vi "Connect.vi"(7 "AMS":T3, 8 "Error In":errorcluster, 10 "Timeout":i32=5000, 11 "Router":string="127.0.0.1") -> (0 "Error Out":errorcluster, 1 "Device Name":string, 2 "ADS Error":T1 items=["NoError"=0, "InternalError"=1, "NoRTime"=2, "LockedMemoryError"=3, "MailBoxError"=4, "WrongHMsg"=5, "TargetPortNotFound"=6, "TargetMachineNotFound"=7, "UnknownCommandID"=8, "BadTaskID"=9, "NoIO"=10, "UnknownAmsCommand"=11, "Win32Error"=12, "PortNotConnected"=13, "InvalidAmsLength"=14, "InvalidAmsNetID"=15, "AmsSyncAmsError"=22, "AmsSyncNoIndexMap"=23, "InvalidAmsPort"=24, "NoMemory"=25, "TCPSendError"=26, "HostUnreachable"=27, "NoLockedMemory"=1280, "MailboxFull"=1282, "DeviceError"=1792, "DeviceServiceNotSupported"=1793, "DeviceInvalidGroup"=1794, "DeviceInvalidOffset"=1795, "DeviceInvalidAccess"=1796, "DeviceInvalidSize"=1797, "DeviceInvalidData"=1798, "DeviceNotReady"=1799, "DeviceBusy"=1800, "DeviceInvalidContext"=1801, "DeviceNoMemory"=1802, "DeviceInvalidParam"=1803, "DeviceNotFound"=1804, "DeviceSyntaxError"=1805, "DeviceIncompatible"=1806, "DeviceExists"=1807, "DeviceSymbolNotFound"=1808, "DeviceSymbolVersionInvalid"=1809, "DeviceInvalidState"=1810, "DeviceTransModeNotSupported"=1811, "DeviceNotifyHandleInvalid"=1812, "DeviceClientUnknown"=1813, "DeviceNoMoreHandles"=1814, "DeviceInvalidWatchsize"=1815, "DeviceNotInitialized"=1816, "DeviceTimeOut"=1817, "DeviceNoInterface"=1818, "DeviceInvalidInterface"=1819, "DeviceInvalidCLSID"=1820, "DeviceInvalidObjectID"=1821, "ClientError"=1856, "ClientInvalidParameter"=1857, "ClientListEmpty"=1858, "ClientVariableInUse"=1859, "ClientDuplicateInvokeID"=1860, "ClientSyncTimeOut"=1861, "ClientW32OR"=1862, "ClientTimeoutInvalid"=1863, "ClientPortNotOpen"=1864, "ClientNoAmsAddr"=1865, "ClientSyncInternal"=1872, "ClientAddHash"=1873, "ClientRemoveHash"=1874, "ClientNoMoreSymbols"=1875, "ClientSyncResInvalid"=1876, "ClientSyncPortLocked"=1877, "ClientQueueFull"=1878], 3 "AMS Connection":T2)   [LabVIEW 2020, in "TwinCAT ADS.lvlib"]
doc: "This connects to the <b>Router</b> (meaning any ADS server, defaults to localhost) via TCP and returns the Device Name for the <b>Target Net ID</b> and <b>Target Port</b> as well as any returned <b>ADS Error</b>. The connection may be established beside of an ADS Error."
uses:
  <userlib>/PMA/TwinCAT ADS.lvlib
  <userlib>/PMA/Low Level/TypeDefs/AMS.ctl
  <userlib>/PMA/Low Level/TypeDefs/AMS Connection.ctl
  <userlib>/PMA/Low Level/TypeDefs/ADS Error.ctl
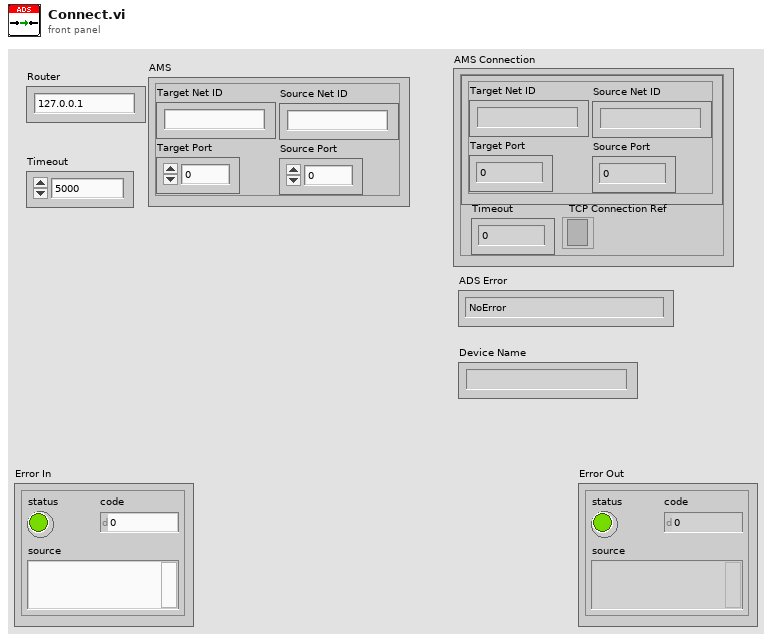
[diagram p1: front panel]
types:
  T1 = typedef "TwinCAT ADS.lvlib/ADS Error.ctl" = i32
  T2 = typedef "TwinCAT ADS.lvlib/AMS Connection.ctl" = cluster{"AMS":T3, "Timeout":i32, "TCP Connection Ref":refnum<k5>}
  T3 = typedef "TwinCAT ADS.lvlib/AMS.ctl" = cluster{"Target Net ID":string, "Target Port":u16, "Source Net ID":string, "Source Port":u16}
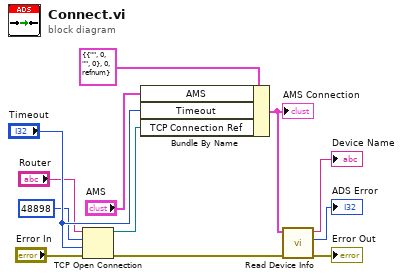
[diagram p0: block diagram]
diagram:
  n1 = TCP Open Connection(address="Router", remote port or service name=u16 48898, timeout ms (60000)="Timeout", error in (no error)="Error In") -> (connection ID=w6:refnum<k5>, error out=w5:errorcluster)  [unwired: 1 in]
  n2 = Bundle By Name(cluster=T2 {"AMS"={"Target Net ID"="", "Target Port"=0, "Source Net ID"="", "Source Port"=0}, "Timeout"=0, "TCP Connection Ref"=refnum} ("AMS Connection"), "AMS"="AMS", "Timeout"="Timeout", "TCP Connection Ref"=w6) -> (w1:T2)
  "AMS Connection" <- w1
  n3 = call <userlib>:"Read Device Info.vi"("Error In"=w5, "AMS Connection In"=w1) -> ("Error Out"=→"Error Out":errorcluster, "ADS Error"=→"ADS Error":T1, "Device Name"=→"Device Name":string)  [unwired: 6 in, 1 out]
